vi "Splite Reason String Part.vi"(7 "Single-line -& Reason":string) -> (4 "CSM Name":string, 8 "`State":string, 15 "`Arguments":string)   [LabVIEW 2017, in "Communicable State Machine.lvlib"]
doc: "-- <b>Controls</b> --\n- <b>Single-line -& Reason</b>:\n\n-- <b>Indicators</b> --\n- <b>CSM Name</b>:\n- <b>`State</b>:\n- <b>`Arguments</b>:"
uses:
  Communicable State Machine.lvlib
  _Shared/CSM Shared.lvlib
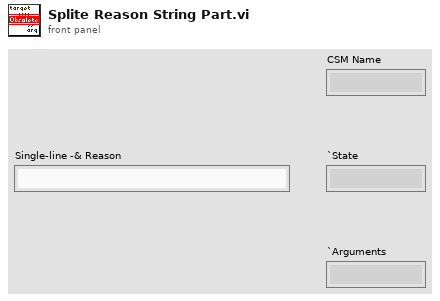
[diagram p1: front panel]
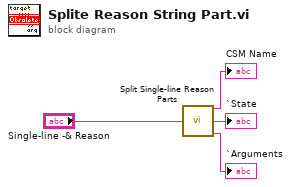
[diagram p0: block diagram]
diagram:
  n1 = call "Split Single-line Reason Parts.vi"("Single-line -& Reason"="Single-line -& Reason") -> ("CSM Name"=→"CSM Name":string, "`State"=→"`State":string, "`Arguments"=→"`Arguments":string)  [unwired: 12 in]
